vi "Get resolution.vi"(0 "Zaber in":T1={"Serial port handle"="", "Axis"="", "Controller #"=0, "Min position"=0.0, "Max position"=0.0, "Min velocity"=0.0, "Max velocity"=0.0, "Firmware"="", "Device ID"=0, "Variable event"=refnum, "Variable ref"=refnum, "Resolution, usteps/step"=0, "Serial port semaphore"=refnum, "Joystick buttons"={"MinDir"=1, "MaxDir"=2, "MedSpeed"=5, "HighSpeed"=6}} {"Joystick buttons"."HighSpeed" min=1 max=25 step=1; "Joystick buttons"."MedSpeed" min=1 max=25 step=1; "Joystick buttons"."MaxDir" min=1 max=25 step=1; "Joystick buttons"."MinDir" min=1 max=25 step=1}, 5 "error in":errorcluster) -> (14 "Zaber out":T1={"Serial port handle"="", "Axis"="", "Controller #"=0, "Min position"=0.0, "Max position"=0.0, "Min velocity"=0.0, "Max velocity"=0.0, "Firmware"="", "Device ID"=0, "Variable event"=refnum, "Variable ref"=refnum, "Resolution, usteps/step"=0, "Serial port semaphore"=refnum, "Joystick buttons"={"MinDir"=1, "MaxDir"=2, "MedSpeed"=5, "HighSpeed"=6}} {"Joystick buttons"."HighSpeed" min=1 max=25 step=1; "Joystick buttons"."MedSpeed" min=1 max=25 step=1; "Joystick buttons"."MaxDir" min=1 max=25 step=1; "Joystick buttons"."MinDir" min=1 max=25 step=1}, 16 "Resolution, usteps/step":u16, 19 "error out":errorcluster)   [LabVIEW 2018]
uses:
  Zaber.ctl
  GenericDataEvent/GenericEvent.ctl
  ZaberVariables.ctl
  CommandZaber.ctl
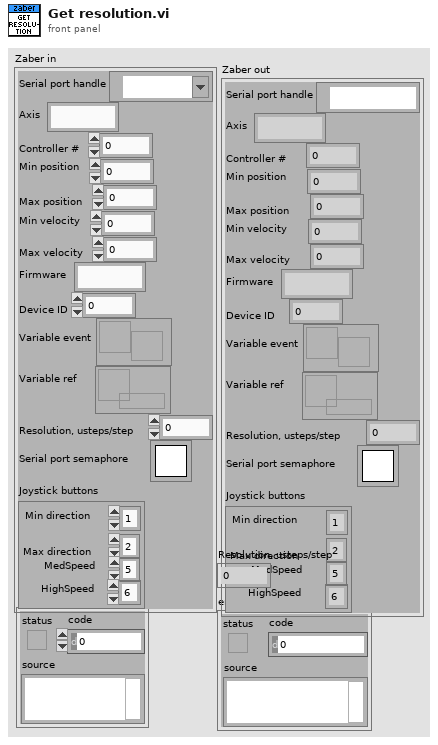
[diagram p1: front panel]
types:
  T1 = typedef "Zaber.ctl" = cluster{"Serial port handle":refnum<visa-resource-name>, "Axis":string, "Controller #":u8, "Min position":dbl, "Max position":dbl, "Min velocity":dbl, "Max velocity":dbl, "Firmware":string, "Device ID":i32, "Variable event":T2, "Variable ref":refnum<data-value>, "Resolution, usteps/step":i32, "Serial port semaphore":T3, "Joystick buttons":cluster{"MinDir":i32, "MaxDir":i32, "MedSpeed":i32, "HighSpeed":i32}}
  T2 = typedef "GenericEvent.ctl" = refnum<user-event>
  T3 = typedef "Semaphore RefNum" = refnum<k1>
  T4 = typedef "CommandZaber.ctl" = cluster{"Command":u8, "Data":i32}
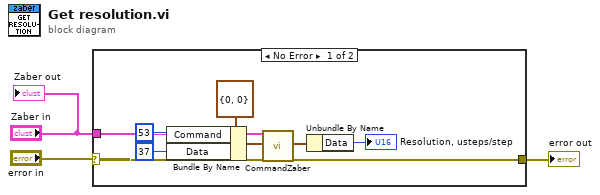
[diagram p0: block diagram]
diagram:
  n1 = case shown="No Error" "error in" {
    selector: "error in" -> [w7 w13]
    tunnel: [w4 w13] -> w2
    tunnel: "Zaber in" -> [w6 _]
    frame No Error {
      n2 = Bundle By Name(cluster=T4 {"Command"=0, "Data"=0} ("Command"), "Command"=53 ("Data"), "Data"=37) -> (w11:T4)
      n3 = call "CommandZaber.vi"("Zaber"=w6, "Command"=w11, "error in"=w7) -> ("Answer"=w8:T4, "error out"=w4:errorcluster)  [unwired: 13 in, 2 out]
      n4 = Unbundle By Name(w8) -> ("Data"=→"Resolution, usteps/step":i32)
    }
    frame Error {
    }
  }
  "error out" <- w2
  "Zaber out" <- "Zaber in"
